vi "Actor Core.vi"(8 "error in":errorcluster, 11 "Game State":refnum<class "Game State.lvclass">) -> (0 "error out":errorcluster, 3 "Actor out":refnum<class "Actor.lvclass">)   [LabVIEW 2021, in "Game State Actor.lvlib" / "Game State.lvclass"]
doc: "This is Actor Core.vi, the main message handling loop for Actors. An actor usually just sits in this loop and processes messages as they arrive. Any error returned by the message Do.vi call will stop the loop, with error code 43 as the canonical signal to stop with no error sent to caller. Descendants may override that in Handle Error.vi."
uses:
  Game State.lvclass
  C:/Program Files (x86)/National Instruments/LabVIEW 2021/vi.lib/ActorFramework/Actor/Actor.lvclass
  <vilib>/ActorFramework/Actor/Actor.lvclass
  <vilib>/ActorFramework/Actor/Actor.lvclass/Actor.ctl
  <vilib>/ActorFramework/Message Enqueuer/Message Enqueuer.lvclass/Message Enqueuer.ctl
  Game State.lvclass/Game State.ctl
  <vilib>/ActorFramework/Message Enqueuer/Init from Existing Queue.vi
  Game State Task Msg/Game State Task Msg.lvclass
  C:/Program Files (x86)/National Instruments/LabVIEW 2021/vi.lib/ActorFramework/Message/Message.lvclass
  <vilib>/ActorFramework/Message Enqueuer/Message Enqueuer.lvclass
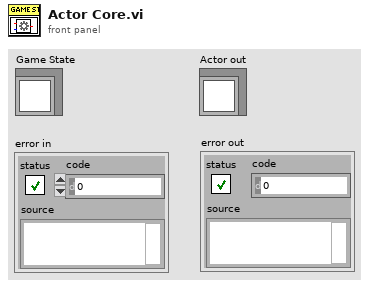
[diagram p1: front panel]
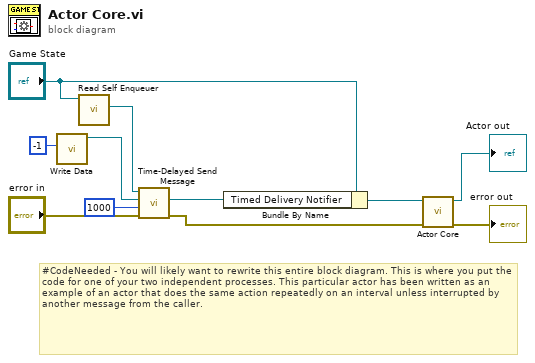
[diagram p0: block diagram]
diagram:
  # "#CodeNeeded - You will likely want to rewrite this entire block diagram. This is where you put the code for one of your two independent processes. This particular actor has been written as an example of an actor that does the same action repeatedly on an interval unless interrupted by another message from the caller."
  n1 = call "Write Data.vi"("Data"=-1) -> ("Game State Task Msg out"=w2:refnum<class "Game State Task Msg.lvclass">)  [unwired: 10 in]
  n2 = call <vilib>:"Read Self Enqueuer.vi"("Actor"="Game State") -> ("Self Enqueuer"=w9:refnum<class "Message Enqueuer.lvclass">)  [unwired: 10 in]
  n3 = call <vilib>:"Time-Delayed Send Message.vi"("error in (no error)"="error in", "Milliseconds To Wait"=1000, "Message"=w2, "Message Enqueuer"=w9) -> ("error out"=w3:errorcluster, "Delivery Notifier"=w5:refnum<notifier>)  [unwired: 6 in]
  n4 = Bundle By Name(cluster="Game State", "Timed Delivery Notifier"=w5) -> (w6:refnum<class "Game State.lvclass">)
  n5 = call-parent "Actor Core.vi"("error in"=w3, "Actor in"=w6) -> ("error out"=→"error out":errorcluster, "Actor out"=→"Actor out":refnum<class "Actor.lvclass">)  [unwired: 8 in]
